vi "Slow Rate.vi"(8 "error in (no error)":errorcluster, 11 "SwipeScrollListbox in":refnum<class "SwipeScrollListbox.lvclass">) -> (0 "error out":errorcluster, 3 "SwipeScrollListbox out":refnum<class "SwipeScrollListbox.lvclass">)   [LabVIEW 2020, in "SwipeScrollListbox.lvclass"]
uses:
  SwipeScrollListbox.lvclass
  SwipeScrollListbox.lvclass/SwipeScrollListbox.ctl
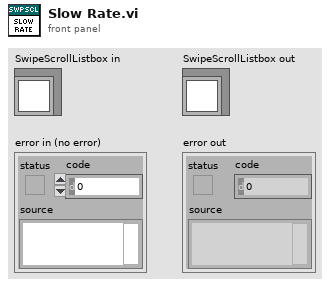
[diagram p1: front panel]
types:
  T1 = typedef "SwipeScrollListbox.lvclass/State Data.ctl" = cluster{"Timeout":i32, "Time":timestamp, "Y":i32, "Slow Distance":i32, "Rate":dbl, "Row Selected":i32}
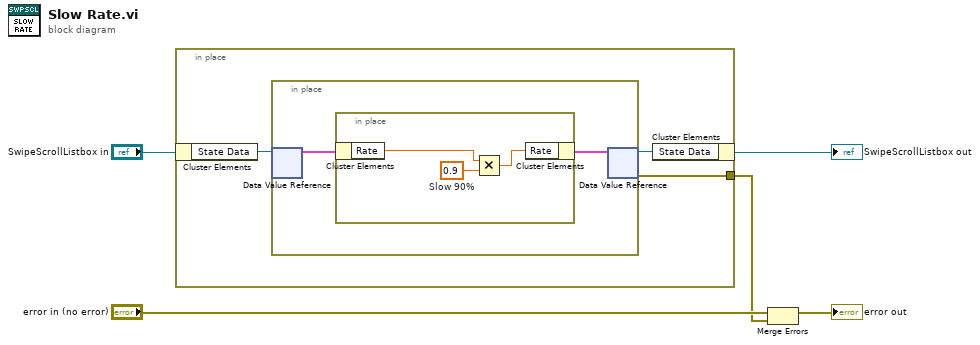
[diagram p0: block diagram]
diagram:
  n1 = in-place {
    in-place-border: [w6] -> w1
    n2 = in-place-cluster #1("SwipeScrollListbox in") -> ("State Data"=w8:refnum<data-value>)
    n3 = in-place {
      n4 = in-place-dvr #2(w8) -> (w10:T1)  [unwired: 1 out]
      n5 = in-place {
        w13 = 0.9  # Slow 90%
        n6 = in-place-cluster #3(w10) -> ("Rate"=w12:dbl)
        n7 = Multiply(x=w12, y=w13) -> (x*y=w11:dbl)
        n8 = in-place-cluster #3("Rate"=w11) -> (w9:T1)
      }
      n9 = in-place-dvr #2(w9) -> (w7:refnum<data-value>, w6:errorcluster)
    }
    n10 = in-place-cluster #1("State Data"=w7) -> (→"SwipeScrollListbox out":refnum<class "SwipeScrollListbox.lvclass">)
  }
  n11 = Merge Errors("error in (no error)", w1) -> (→"error out":errorcluster)
